vi "Load_Zspec_param_options.vi"(10 "Zspecparam.txt location":path, 11 "Array in":refnum<vi>) -> (1 "Array":string[](array[string]), 2 "Zspec Types []":string[](array[string]), 3 "data\n\n 4":T1(array[cluster]))   [LabVIEW 2014]
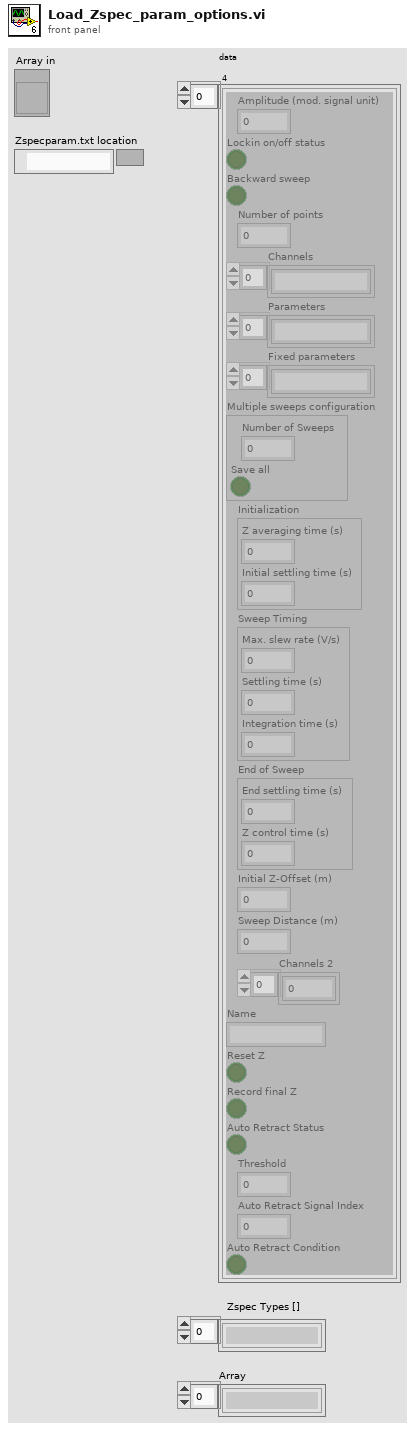
[diagram p1: front panel]
types:
  T1 = cluster{"Amplitude (mod. signal unit)":sgl, "Lockin on/off status":bool, "Backward sweep":bool, "Number of points":i32, "Channels":string[], "Parameters":string[], "Fixed parameters":string[], "Multiple sweeps configuration":cluster{"Number of Sweeps":i32, "Save all":bool}, "Initialization":cluster{"Z averaging time (s)":sgl, "Initial settling time (s)":sgl}, "Sweep Timing":cluster{"Max. slew rate (V/s)":sgl, "Settling time (s)":sgl, "Integration time (s)":sgl}, "End of Sweep":cluster{"End settling time (s)":sgl, "Z control time (s)":sgl}, "Initial Z-Offset (m)":sgl, "Sweep Distance (m)":sgl, "Channels 2":i32[], "Name":string, "Reset Z":bool, "Record final Z":bool, "Auto Retract Status":bool, "Threshold":sgl, "Auto Retract Signal Index":i32, "Auto Retract Condition":bool}[]
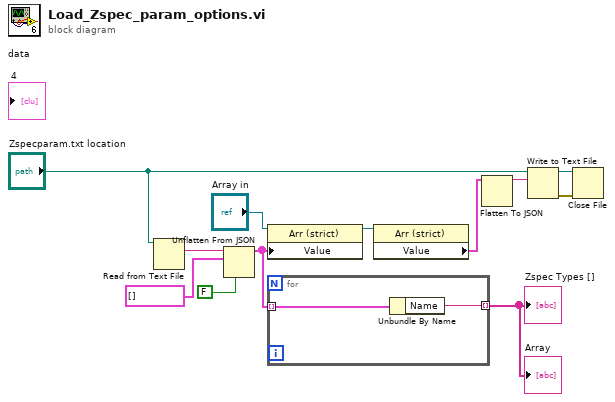
[diagram p0: block diagram]
diagram:
  n1 = Read from Text File(file (use dialog)="Zspecparam.txt location") -> (text=w8:string)  [unwired: 3 in, 3 out]
  n2 = Unflatten From JSON(JSON string=w8, type and defaults=T1 [] ("data"), default null elements? (F)=FALSE) -> (value=w12:T1)  [unwired: 4 in, 1 out]
  n3 = property class="Arr (strict)"(reference="Array in", "Value"=w12) -> (reference out=w1:refnum<vi>)  [unwired: 1 in, 1 out]
  n4 = for {
    tunnel: w12 -> [w14] mode=indexing
    tunnel: [w13] -> w10 mode=indexing
    n5 = Unbundle By Name(w14) -> ("Name"=w13:string)
  }
  "Zspec Types []" <- w10
  "Array" <- w10
  n6 = property class="Arr (strict)"(reference=w1) -> ("Value"=w11:T1)  [unwired: 1 in, 2 out]
  n7 = Flatten To JSON(anything=w11) -> (JSON string=w5:string)  [unwired: 2 in, 1 out]
  n8 = Write to Text File(file (use dialog)="Zspecparam.txt location", text=w5) -> (refnum out=w3:refnum<file>, error out=w4:errorcluster)  [unwired: 2 in, 1 out]
  n9 = Close File(refnum=w3, error in=w4) -> ()  [unwired: 2 out]
